vi "hadec2altaz.vi"(9 "LAT":dbl format="%.6g", 10 "DEC":dbl, 11 "HA":dbl) -> (1 "Gz":dbl, 2 "Gy":dbl, 3 "Gx":dbl, 4 "Alt (theta)":dbl, 6 "Az (phi)":dbl)   [LabVIEW 2011]
panel:
  out "R":dbl
  out "r":dbl
  out "z":dbl
  out "y":dbl
  out "x":dbl
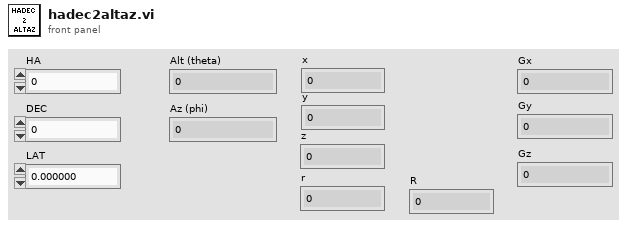
[diagram p1: front panel]
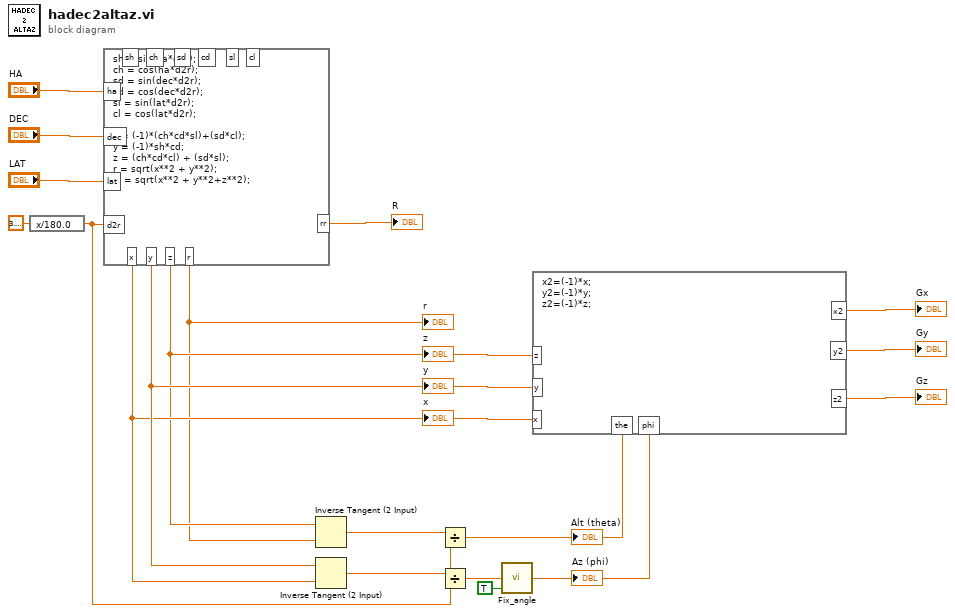
[diagram p0: block diagram]
diagram:
  n1 = expression code="x/180.0"(3.141592653589793) -> (w9:dbl)
  n2 = formula code="sh = sin(ha*d2r);\nch = cos(ha*d2r);\nsd = sin(dec*d2r);\ncd = cos(dec*d2r);\nsl = sin(lat*d2r);\ncl = cos(lat*d2r);\n\nx = (-1)*(ch*cd*sl)+(sd*cl);\ny = (-1)*sh*cd;\nz = (ch*cd*cl) + (sd*sl);\nr = sqrt(x**2 + y**2);\nrr = sqrt(x**2 + y**2+z**2);"("ha"="HA", "dec"="DEC", "lat"="LAT", "d2r"=w9) -> ("x"=w14:dbl, "y"=w15:dbl, "z"=w12:dbl, "r"=w11:dbl, "rr"=→"R":dbl)  [unwired: 6 out]
  "x" <- w14
  "y" <- w15
  "z" <- w12
  "r" <- w11
  n3 = Inverse Tangent (2 Input)(1:w11, 2:w12) -> (0:w10:dbl)
  n4 = Inverse Tangent (2 Input)(1:w14, 2:w15) -> (0:w13:dbl)
  n5 = Divide(x=w10, y=w9) -> (x/y=w6:dbl)
  "Alt (theta)" <- w6
  n6 = Divide(x=w13, y=w9) -> (x/y=w7:dbl)
  n7 = call "Fix_angle.vi"("±180 -> 0-360?"=TRUE, "Angle IN"=w7) -> ("Angle OUT"=w5:dbl)  [unwired: 3 in]
  "Az (phi)" <- w5
  n8 = formula code="x2=(-1)*x;\ny2=(-1)*y;\nz2=(-1)*z;"("x"=w14, "y"=w15, "z"=w12, "the"=w6, "phi"=w5) -> ("x2"=→"Gx":dbl, "y2"=→"Gy":dbl, "z2"=→"Gz":dbl)
